vi "PCO_ConvertDelete.vi"(8 "error in (no error)":errorcluster {"code" format="%x"}, 11 "ph":u64) -> (0 "error out":errorcluster {"code" format="%x"}, 2 "ErrorMessage":i32 format="%x")   [LabVIEW 2020, in "Convert.lvlib"]
doc: "int PCOCONVERT_API PCO_ConvertDelete(HANDLE ph);"
uses:
  Convert.lvlib
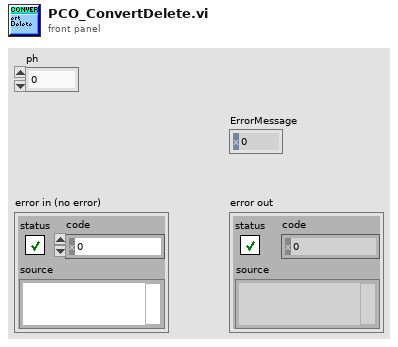
[diagram p1: front panel]
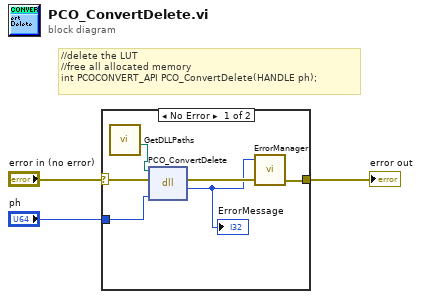
[diagram p0: block diagram]
diagram:
  # "//delete the LUT \n//free all allocated memory\nint PCOCONVERT_API PCO_ConvertDelete(HANDLE ph);"
  n1 = case shown="No Error" "error in (no error)" {
    selector: "error in (no error)" -> [w5 w10]
    tunnel: "ph" -> [w9 _]
    tunnel: [w7 w10] -> w2
    frame No Error {
      n2 = call "GetDLLPaths.vi"() -> ("PCO_Conv_Path"=w4:path)  [unwired: 9 in, 2 out]
      n3 = dll-call lib="?" fn="PCO_ConvertDelete"(path in=w4, error in=w5, "ph"=w9) -> (error out=w8:errorcluster, "return type"=w6:i32)  [unwired: 2 in, 1 out]
      "ErrorMessage" <- w6
      n4 = call "ErrorManager.vi"("error in (no error)"=w8, "error code"=w6) -> ("error out"=w7:errorcluster)  [unwired: 3 in]
    }
    frame Error {
    }
  }
  "error out" <- w2
